vi "take_derivative_subvi.vi"(10 "X in":waveform(dbl), 11 "sampling info":cluster{"Fs":dbl, "#s":dbl}) -> (0 "index of max":dbl, 1 "X out":waveform(dbl), 2 "derivative out":waveform(dbl), 3 "max peak height":dbl)   [LabVIEW 2015]
uses:
  <vilib>/Analysis/3filter.llb/Filter Passband Type.ctl
  <vilib>/Analysis/3filter.llb/Butterworth Filter (DBL).vi
  <vilib>/Analysis/NI_AALPro.lvlib
  <vilib>/Analysis/NI_AALBase.lvlib
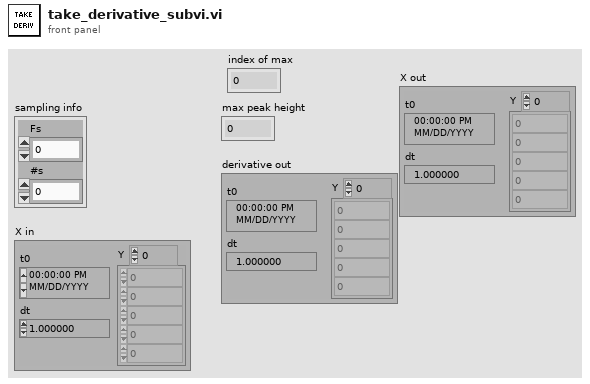
[diagram p1: front panel]
types:
  T1 = typedef "NI_AALBase.lvlib/Filter Passband Type.ctl" = enum32{"Lowpass", "Highpass", "Bandpass", "Bandstop"}
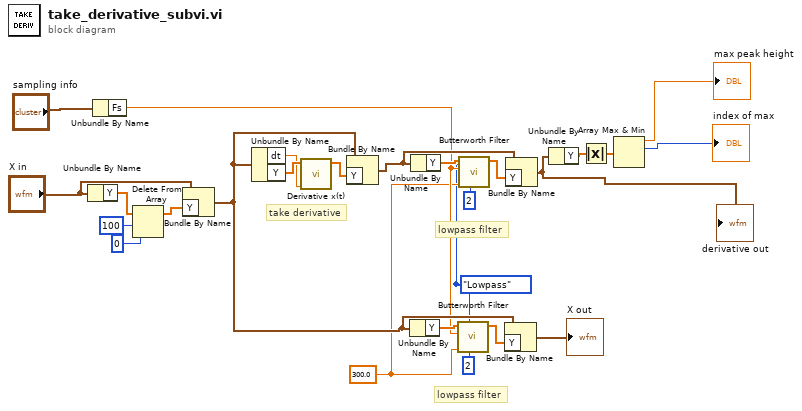
[diagram p0: block diagram]
diagram:
  w1 = Filter_Passband_Type."Lowpass" ("filter type")
  w5 = 300.0 ("low cutoff freq: fl")
  # "lowpass filter"
  # "lowpass filter"
  # "take derivative"
  n1 = Unbundle By Name("X in") -> ("Y"=w15:dbl[])
  n2 = Unbundle By Name("sampling info") -> ("Fs"=w6:dbl)
  n3 = Delete From Array(array=w15, length=100, index=0) -> (array with subset deleted=w14:dbl[])  [unwired: 1 out]
  n4 = Bundle By Name(cluster="X in", "Y"=w14) -> (w8:waveform(dbl))
  n5 = Unbundle By Name(w8) -> ("dt"=w18:dbl, "Y"=w19:dbl[])
  n6 = call <vilib>:"Derivative x(t).vi"("dt"=w18, "X"=w19) -> ("dX/dt"=w17:dbl[])  [unwired: 8 in, 1 out]
  n7 = Bundle By Name(cluster=w8, "Y"=w17) -> (w23:waveform(dbl))
  n8 = Unbundle By Name(w8) -> ("Y"=w9:dbl[])
  n9 = Unbundle By Name(w23) -> ("Y"=w20:dbl[])
  n10 = call-poly <vilib>:"Butterworth Filter.vi"("order"=2, "filter type"=w1, "low cutoff freq: fl"=w5, "sampling freq: fs"=w6, "X"=w9) -> ("Filtered X"=w10:dbl[])  [unwired: 3 in, 1 out]
  n11 = call-poly <vilib>:"Butterworth Filter.vi"("order"=2, "filter type"=w1, "low cutoff freq: fl"=w5, "sampling freq: fs"=w6, "X"=w20) -> ("Filtered X"=w21:dbl[])  [unwired: 3 in, 1 out]
  n12 = Bundle By Name(cluster=w8, "Y"=w10) -> (→"X out":waveform(dbl))
  n13 = Bundle By Name(cluster=w23, "Y"=w21) -> (w25:waveform(dbl))
  "derivative out" <- w25
  n14 = Unbundle By Name(w25) -> ("Y"=w3:dbl[])
  n15 = Absolute Value(x=w3) -> (abs(x)=w2:dbl[])
  n16 = Array Max & Min(array=w2) -> (max value=→"max peak height":dbl, max index (indices)=→"index of max":i32)  [unwired: 2 out]
